vi "ziList.vi"(3 "Error In":errorcluster, 4 "Flags (None)":T2, 5 "Path (\"\")":string, 6 "Handle In":T1 {"Handle" format="0x%08x"; "Conn" format="0x%08x"}) -> (0 "Error Out":errorcluster, 1 "Nodes":string[](array[string]), 2 "Handle Out":T1 {"Handle" format="0x%08x"; "Conn" format="0x%08x"})   [LabVIEW 2009, in "Zurich Instruments LabOne.lvlib"]
doc: "Returns a list of nodes found at the specified path. The path may contain wild cards so that the rertuned nodes do not necessarily have to have the same parents."
uses:
  <instrlib>/Zurich Instruments LabOne/Zurich Instruments LabOne.lvlib
  <instrlib>/Zurich Instruments LabOne/Public/ziTypeHandle.ctl
  <instrlib>/Zurich Instruments LabOne/Private/ziLV64.dll
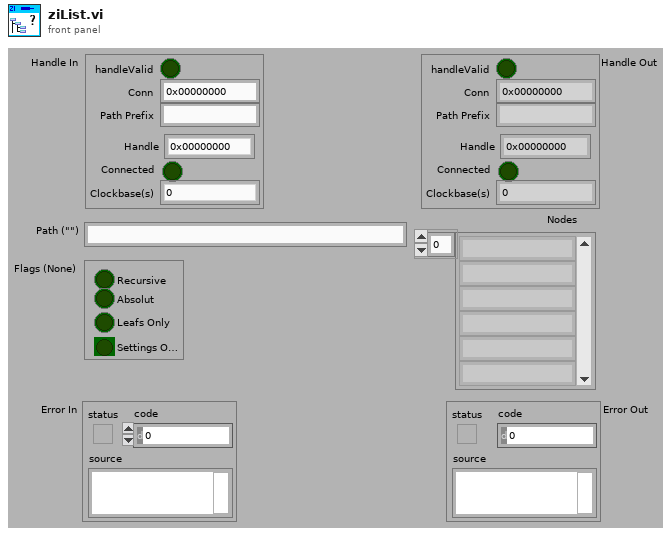
[diagram p1: front panel]
types:
  T1 = typedef "Zurich Instruments LabOne.lvlib/ziTypeHandle.ctl" = cluster{"handleValid":bool, "Conn":u64, "Path Prefix":string, "Handle":u64, "Connected":bool, "Clockbase(s)":dbl}
  T2 = cluster{"Recursive":bool, "Absolut":bool, "Leafs Only":bool, "Settings Only":bool}
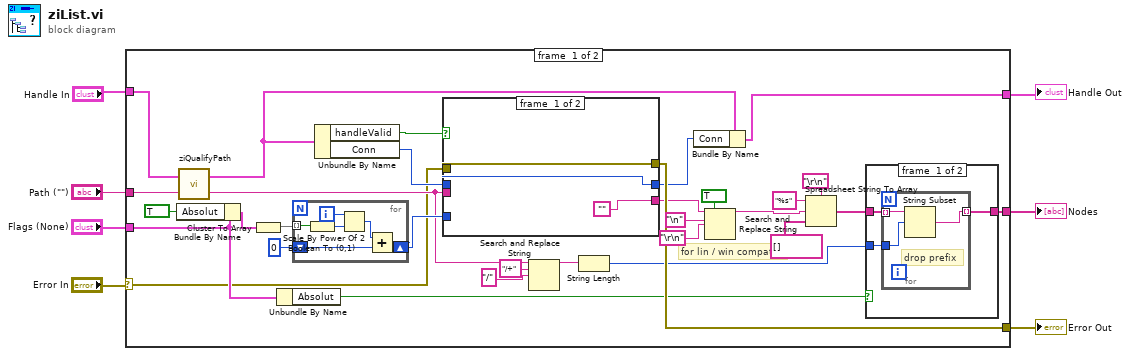
[diagram p0: block diagram]
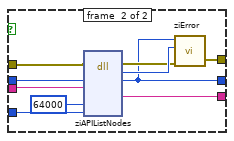
[diagram p3: hidden frame]
diagram:
  n1 = case shown="No Error" "Error In" {
    selector: "Error In" -> [w8 w66]
    tunnel: [w38 w66] -> w7
    tunnel: [w24 w65] -> w6
    tunnel: "Path (\"\")" -> [w23 _]
    tunnel: "Handle In" -> [w22 w65]
    tunnel: "Flags (None)" -> [w19 _]
    tunnel: [w12 _] -> w2
    frame #0 {
      # "for lin / win compat"
      n2 = Bundle By Name(cluster=w19, "Absolut"=TRUE) -> (w18:T2)
      n3 = call <instrlib>:"ziQualifyPath.vi"("Path In"=w23, "Handle In"=w22) -> ("Path Out"=w9:string, "Handle Out"=w21:T1)
      n4 = Cluster To Array(cluster=w18) -> (array=w34:bool[])
      n5 = Unbundle By Name(w19) -> ("Absolut"=w14:bool)
      n6 = for {
        tunnel: w34 -> [w51] mode=indexing
        shift-right: [w47] -> w32
        shift-left: 0 -> [w48]
        i -> [w46]
        n7 = Boolean To (0,1)(Boolean=w51) -> (0, 1=w50:i16)
        n8 = Scale By Power Of 2(n=w46, x=w50) -> (x*2^n=w49:i16)
        n9 = Add(x=w49, y=w48) -> (x+y=w47:i32)
      }
      n10 = Unbundle By Name(w21) -> ("handleValid"=w37:bool, "Conn"=w36:u64)
      n11 = case shown="True" w37 {
        tunnel: ["" w63] -> w28
        tunnel: w8 -> [w53 w61]
        tunnel: w36 -> [w52 w62]
        tunnel: [w52 w55] -> w35
        tunnel: [w53 w56] -> w38
        tunnel: w9 -> [_ w59]
        tunnel: w32 -> [_ w64]
        frame #0 {
        }
        frame #1 {
          n12 = dll-call lib="C:/Program Files/National Instruments/LabVIEW 2009/instr.lib/Zurich Instruments LabOne/Private/ziLV*.*" fn="ziAPIListNodes"(error in=w61, "Conn"=w62, "Path"=w59, "MaxLen"=64000, "Flags"=w64) -> (error out=w57:errorcluster, "return type"=w58:u32, "Conn"=w55:u64, "Nodes"=w63:string)  [unwired: 5 in, 2 out]
          n13 = call <instrlib>:"ziError.vi"("Conn"=w55, "ziErrorCode"=w58, "Error In"=w57) -> ("Error Out"=w56:errorcluster)  [unwired: 2 in, 1 out]
        }
      }
      n14 = Search and Replace String(input string=w9, search string="/+" ("replace string (\"\")"), replace string="/" ("replace string (\"\")")) -> (result string=w15:string)  [unwired: 2 in, 6 out]
      n15 = String Length(string=w15) -> (length=w11:i32)
      n16 = Bundle By Name(cluster=w21, "Conn"=w35) -> (w24:T1)
      n17 = Search and Replace String(replace all?=TRUE ("replace all? (F)"), input string=w28, search string="\n", replace string="\r\n") -> (result string=w10:string)  [unwired: 1 in, 6 out]
      n18 = Spreadsheet String To Array(delimiter (Tab)="\r\n", format string="%s", spreadsheet string=w10, array type (2D Dbl)=string[] []) -> (array=w13:string[])
      n19 = case shown="False" w14 {
        tunnel: w13 -> [w41 w45]
        tunnel: [w40 w45] -> w12
        tunnel: w11 -> [w39 _]
        frame #0 {
          n20 = for {
            tunnel: w41 -> [w44] mode=indexing
            tunnel: [w43] -> w40 mode=indexing
            tunnel: w39 -> [w42]
            # "drop prefix"
            n21 = String Subset(string=w44, offset (0)=w42) -> (substring=w43:string)  [unwired: 1 in]
          }
        }
        frame #1 {
        }
      }
    }
    frame #1 {
    }
  }
  "Error Out" <- w7
  "Nodes" <- w2
  "Handle Out" <- w6
